vi "Load Config.vi"(8 "error in (no error)":errorcluster, 10 "Config Path":path, 11 "Editor in":refnum<class "Editor.lvclass">) -> (0 "error out":errorcluster, 3 "Editor out":refnum<class "Editor.lvclass">)   [LabVIEW 2020, in "VolatusGUIEditor.lvlib" / "Editor.lvclass"]
uses:
  Editor.lvclass
  Editor.lvclass/Editor.ctl
  lv-volatus/VolatusConfig/VolatusConfig/VolatusConfig.lvclass
  lv-volatus/VolatusConfig/VolatusConfig.lvlib
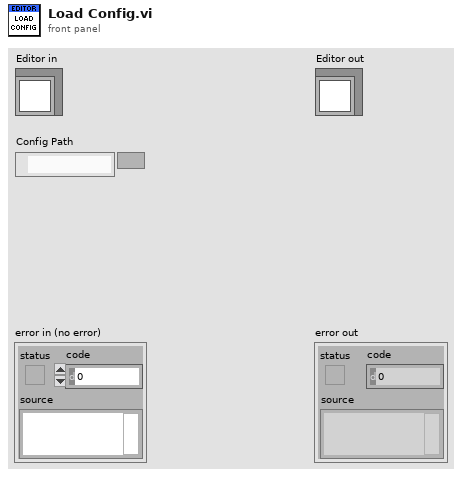
[diagram p1: front panel]
types:
  T1 = typedef "VolatusConfig.lvlib/Config Format.ctl" = enum16{"JSON", "INI", "SQLite"}
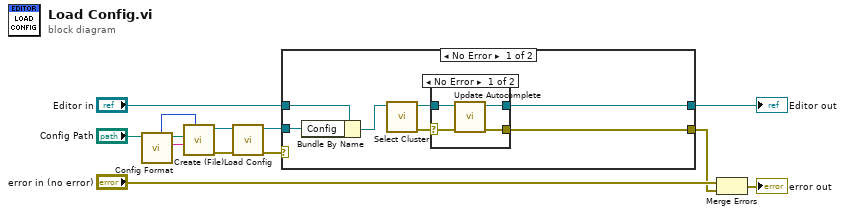
[diagram p0: block diagram]
diagram:
  n1 = call "Config Format.vi"("Config Path"="Config Path") -> ("filename without extension"=w10:string, "Folder"=w11:path, "Format"=w12:T1)  [unwired: 8 in]
  n2 = call "Create (File).vi"("Main Format"=w12, "Main Filename"=w10, "Config Root"=w11) -> ("error out"=w7:errorcluster, "VolatusConfig out"=w8:refnum<class "VolatusConfig.lvclass">)  [unwired: 7 in]
  n3 = call "Load Config.vi"("error in (no error)"=w7, "VolatusConfig in"=w8) -> ("error out"=w5:errorcluster, "VolatusConfig out"=w4:refnum<class "VolatusConfig.lvclass">)  [unwired: 7 in, 1 out]
  n4 = case shown="No Error" w5 {
    selector: w5 -> [_ w28]
    tunnel: "Editor in" -> [w20 w27]
    tunnel: w4 -> [w19 _]
    tunnel: [w17 w27] -> w3
    tunnel: [w16 w28] -> w1
    frame No Error {
      n5 = Bundle By Name(cluster=w20, "Config"=w19) -> (w18:refnum<class "Editor.lvclass">)
      n6 = call "Select Cluster.vi"("Editor in"=w18) -> ("error out"=w14:errorcluster, "Editor out"=w15:refnum<class "Editor.lvclass">)  [unwired: 9 in]
      n7 = case shown="No Error" w14 {
        selector: w14 -> [w21 w25]
        tunnel: [w24 w26] -> w17
        tunnel: [w23 w25] -> w16
        tunnel: w15 -> [w22 w26]
        frame No Error {
          n8 = call "Update Autocomplete.vi"("error in (no error)"=w21, "Editor in"=w22) -> ("error out"=w23:errorcluster, "Editor out"=w24:refnum<class "Editor.lvclass">)  [unwired: 8 in]
        }
        frame Error {
        }
      }
    }
    frame Error {
    }
  }
  "Editor out" <- w3
  n9 = Merge Errors("error in (no error)", w1) -> (→"error out":errorcluster)
